vi "IPS Reply to PGSQL.vi"(8 "error in (no error)":errorcluster, 10 "Response":T1, 11 "Instrument.1820 in":refnum<class "Instrument.OxfordVRM.lvclass">) -> (0 "error out":errorcluster, 3 "Instrument.1820 out":refnum<class "Instrument.OxfordVRM.lvclass">)   [LabVIEW 2016, in "Instrument.OxfordVRM.lvclass"]
uses:
  Instrument.OxfordVRM.lvclass
  <instrlib>/Mercury iXX/Public/Controls/Response String.ctl
  <userlib>/LevyLab/Levylab Instruments/SMOs/Logger.PGSQL/Logger.PGSQL.lvclass
  <userlib>/LevyLab/Levylab Instruments/SMOs/Instrument/Instrument.lvclass
  C:/Program Files (x86)/National Instruments/LabVIEW 2016/user.lib/LevyLab/Levylab Instruments/SMOs/Instrument/Instrument.lvclass
  <instrlib>/Mercury iXX/Mercury iXX.lvlib
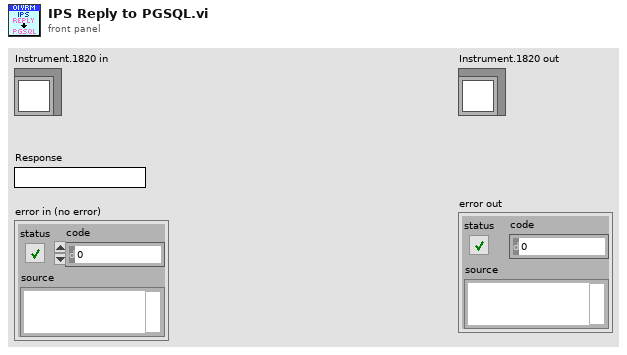
[diagram p1: front panel]
types:
  T1 = typedef "Mercury iXX.lvlib/Response String.ctl" = string
  T2 = cluster{"RemoteControl":refnum<class "RemoteControl.lvclass">, "Logger.DSC":refnum<class "Logger.DSC.lvclass">, "Logger.Error":refnum<class "Logger.Error.lvclass">, "Logger.PGSQL":refnum<class "Logger.PGSQL.lvclass">}
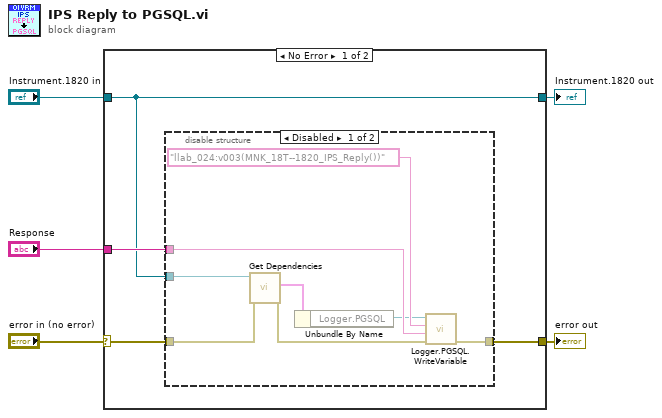
[diagram p0: block diagram]
diagram:
  n1 = case shown="No Error" "error in (no error)" {
    selector: "error in (no error)" -> [w7 w18]
    tunnel: "Response" -> [w9 _]
    tunnel: [w8 w18] -> w4
    tunnel: "Instrument.1820 in" -> [w6 w19]
    tunnel: [w6 w19] -> w1
    frame No Error {
      n2 = disable-structure shown="Disabled" {
        disable-tunnel: w9 -> [w17 _]
        disable-tunnel: [w15 _] -> w8
        disable-tunnel: w7 -> [w11 _]
        disable-tunnel: w6 -> [w10 _]
        frame Disabled {
          n3 = call <userlib>:"Get Dependencies.vi"("error in (no error)"=w11, "Instrument in"=w10) -> ("error out"=w12:errorcluster, "Dependencies"=w13:T2)  [unwired: 7 in, 1 out]
          n4 = Unbundle By Name(w13) -> ("Logger.PGSQL"=w14:refnum<class "Logger.PGSQL.lvclass">)
          n5 = call <userlib>:"Logger.PGSQL.WriteVariable.vi"("error in (no error)"=w12, "Data"=w17, "Address"="llab_024:v003(MNK_18T--1820_IPS_Reply())" ("variable"), "Logger"=w14) -> ("error out"=w15:errorcluster)  [unwired: 6 in, 1 out]
        }
        frame Enabled {
        }
      }
    }
    frame Error {
    }
  }
  "error out" <- w4
  "Instrument.1820 out" <- w1
